vi "Set_2400_Voltage.vi"(7 "error in":errorcluster, 9 "Voltage":dbl format="%_6g") -> (0 "error out":errorcluster)   [LabVIEW 2020]
uses:
  <instrlib>/Keithley 24XX/Keithley 24XX.lvlib
panel:
  out "Result":string
  out "Error Message":string
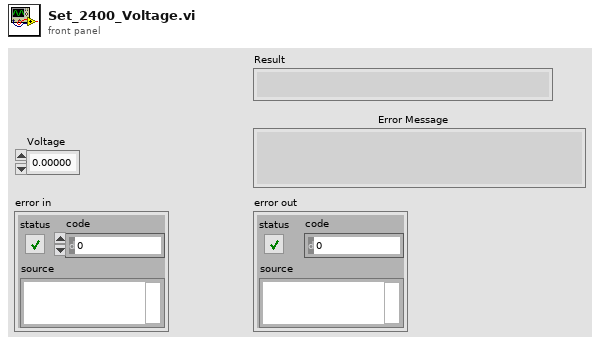
[diagram p1: front panel]
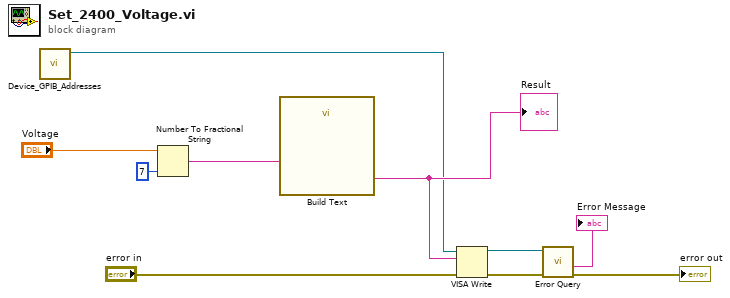
[diagram p0: block diagram]
diagram:
  n1 = call "Device_GPIB_Addresses.vi"() -> ("Keithley 2400 Address"=w8:refnum<visa-resource-name>)  [unwired: 9 in, 2 out]
  n2 = Number To Fractional String(number="Voltage", precision (6)=i16 7) -> (F-format string=w2:string)  [unwired: 2 in]
  n3 = call "Build Text"("VOLTAGE"=w2) -> ("Result"=w10:string)  [unwired: 3 in, 11 out]
  "Result" <- w10
  n4 = VISA Write(VISA resource name=w8, write buffer=w10, error in (no error)="error in") -> (VISA resource name out=w4:refnum<visa-resource-name>, error out=w5:errorcluster)  [unwired: 1 out]
  n5 = call <instrlib>:"Error Query.vi"("error in (no error)"=w5, "VISA resource name"=w4) -> ("error out"=→"error out":errorcluster, "Error Message"=→"Error Message":string)  [unwired: 6 in, 2 out]
